vi "Update speed graph X-scale label.vi"(8 "error in (no error)":errorcluster, 11 "Speed Graph":refnum<vi>) -> (0 "error out":errorcluster)   [LabVIEW 2020]
uses:
  Globals/gl_Time series viewer globals.vi
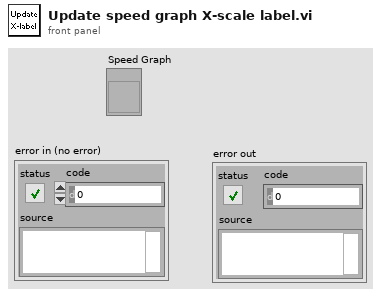
[diagram p1: front panel]
types:
  T1 = typedef "AVI playback header info cluster.ctl" = cluster{"Frame Size":u32, "AOD fill time (us)":dbl, "Dwell time (us)":dbl, "Frame period (ms)":dbl, "Number of Miniscans":u16, "Number of Pixels in Miniscan":u16}
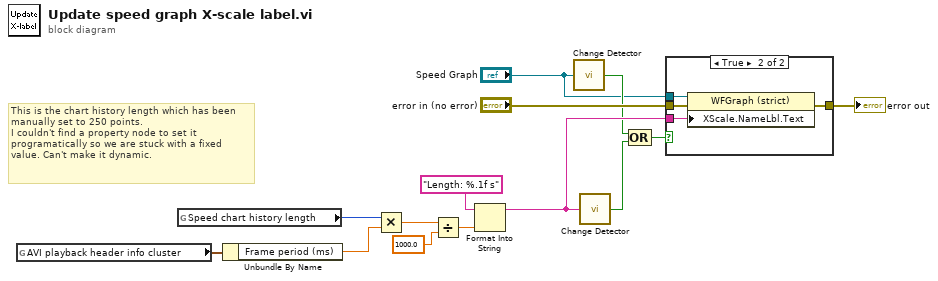
[diagram p0: block diagram]
diagram:
  # "This is the chart history length which has been manually set to 250 points.\nI couldn't find a property node to set it programatically so we are stuck with a fixed value. Can't make it dynamic."
  n1 = global read "gl_Time series viewer globals.vi" "AVI playback header info cluster"() -> (w14:T1)
  n2 = global read "gl_Time series viewer globals.vi" "Speed chart history length"() -> (w10:i32)
  n3 = Unbundle By Name(w14) -> ("Frame period (ms)"=w9:dbl)
  n4 = Multiply(x=w10, y=w9) -> (x*y=w8:dbl)
  n5 = Divide(x=w8, y=1000.0) -> (x/y=w11:dbl)
  n6 = Format Into String(format string="Length: %.1f s", w11) -> (resulting string=w5:string)  [unwired: 2 in, 1 out]
  n7 = call <userlib>:"Change Detector.vi"("Value"="Speed Graph") -> ("Changed?"=w2:bool)
  n8 = call <userlib>:"Change Detector.vi"("Value"=w5) -> ("Changed?"=w3:bool)
  n9 = Compound Arithmetic op=OR(w2, w3) -> (w4:bool)
  n10 = case shown="True" w4 {
    tunnel: "Speed Graph" -> [_ w19]
    tunnel: [w15 w18] -> w7
    tunnel: "error in (no error)" -> [w15 w17]
    tunnel: w5 -> [_ w16]
    frame False {
    }
    frame True {
      n11 = property class="WFGraph (strict)"(reference=w19, error in=w17, "XScale.NameLbl.Text"=w16) -> (error out=w18:errorcluster)  [unwired: 1 out]
    }
  }
  "error out" <- w7
